vi "Read Actual Server Identity.vi"(10 "server errors":string, 11 "client in":refnum<class "PuTTY Client.lvclass">) -> (2 "fingerprint":string, 3 "client out":refnum<class "PuTTY Client.lvclass">)   [LabVIEW 2020, in "NI_SSH.lvlib" / "PuTTY Client.lvclass"]
uses:
  <vilib>/net/SSH/Client/PuTTY/PuTTY Client.lvclass
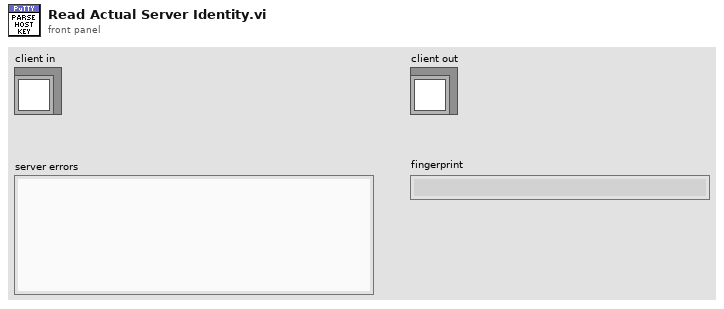
[diagram p1: front panel]
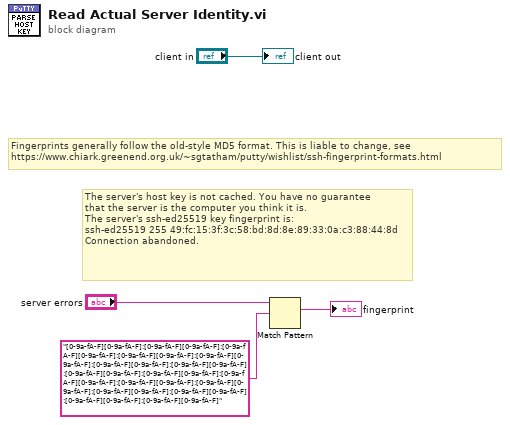
[diagram p0: block diagram]
diagram:
  # "Fingerprints generally follow the old-style MD5 format. This is liable to change, see\nhttps://www.chiark.greenend.org.uk/~sgtatham/putty/wishlist/ssh-fingerprint-formats.html"
  # "The server's host key is not cached. You have no guarantee\nthat the server is the computer you think it is.\nThe server's ssh-ed25519 key fingerprint is:\nssh-ed25519 255 49:fc:15:3f:3c:58:bd:8d:8e:89:33:0a:c3:88:44:8d\nConnection abandoned."
  n1 = Match Pattern(string="server errors", regular expression="[0-9a-fA-F][0-9a-fA-F]:[0-9a-fA-F][0-9a-fA-F]:[0-9a-fA-F][0-9a-fA-F]:[0-9a-fA-F][0-9a-fA-F]:[0-9a-fA-F][0-9a-fA-F]:[0-9a-fA-F][0-9a-fA-F]:[0-9a-fA-F][0-9a-fA-F]:[0-9a-fA-F][0-9a-fA-F]:[0-9a-fA-F][0-9a-fA-F]:[0-9a-fA-F][0-9a-fA-F]:[0-9a-fA-F][0-9a-fA-F]:[0-9a-fA-F][0-9a-fA-F]:[0-9a-fA-F][0-9a-fA-F]:[0-9a-fA-F][0-9a-fA-F]:[0-9a-fA-F][0-9a-fA-F]:[0-9a-fA-F][0-9a-fA-F]") -> (match substring=→"fingerprint":string)  [unwired: 1 in, 3 out]
  "client out" <- "client in"
